vi "Generate Resampling Parameters.vi"(10 "X.ZOOM (Linear)":dbl, 11 "Stretch Array IN":dbl[](array[numeric])=[1.440619470870466, 1.4376467808189701, 1.4346907462529248, 1.431751260882534, 1.4288282193717416, 1.425921517328019, 1.4230310512922835, 1.4201567187289466, 1.4172984180160932, 1.4144560484357853, 1.4116295101644896, 1.4088187042636287, 1.4060235326702533, 1.4032438981878341, 1.4004797044771675, 1.397730856047402, 1.3949972582471741, 1.3922788172558593, 1.3895754400749307, 1.3868870345194306, 1.3842135092095456, 1.3815547735622893, 1.3789107377832892, 1.3762813128586768, 1.3736664105470766, 1.3710659433716992, 1.368479824612527, 1.3659079682986035, 1.3633502892004121, 1.3608067028223534, 1.3582771253953125, 1.3557614738693209, 1.3532596659063045, 1.3507716198729252, 1.348297254833506, 1.3458364905430458, 1.343389247440318, 1.3409554466410527, 1.3385350099312032, 1.3361278597602924, 1.3337339192348416, 1.3313531121118791, 1.328985362792523, 1.3266305963156464, 1.3242887383516175, 1.321959715196112, 1.3196434537640023, 1.3173398815833195, 1.3150489267892873, 1.3127705181184264, 1.3105045849027293, 1.308251057063904, 1.3060098651076884, 1.303780940118227, 1.301564213752519, 1.2993596182349283, 1.2971670863517617, 1.2949865514459058, 1.2928179474115327, 1.2906612086888616, 1.2885162702589879, 1.2863830676387666, 1.2842615368757604, 1.282151614543242, 1.2800532377352587, 1.2779663440617515, 1.2758908716437318, 1.2738267591085115, 1.2717739455849928, 1.2697323706990076, 1.2677019745687121, 1.2656826978000357, 1.2636744814821805, 1.261677267183171, 1.259690996945458, 1.25771561328157, 1.255751059169815, 1.2537972780500308, 1.251854213819384, 1.2499218108282157, 1.248000013875936, 1.2460887682069621, 1.2441880195067057, 1.2422977138976015, 1.2404177979351838, 1.2385482186042058, 1.236688923314801, 1.2348398598986912, 1.233000976605433, 1.2311722220987076, 1.2293535454526525, 1.2275448961482345, 1.2257462240696608, 1.2239574795008314, 1.2221786131218302, 1.2204095760054567, 1.2186503196137932, 1.2169007957948108, 1.2151609567790143, 1.2134307551761225, 1.2117101439717848, 1.2099990765243347, 1.2082975065615775, 1.2066053881776153, 1.204922675829705, 1.2032493243351499, 1.2015852888682272, 1.1999305249571475, 1.1982849884810485, 1.1966486356670185, 1.195021423087156, 1.1934033076556592, 1.1917942466259448, 1.1901941975878023, 1.188603118464577, 1.1870209675103802, 1.1854477033073352, 1.183883284762848, 1.18232767110691, 1.1807808218894282, 1.1792426969775847, 1.1777132565532245, 1.1761924611102694, 1.1746802714521631, 1.1731766486893391, 1.1716815542367196, 1.170194949811237, 1.1687167974293855, 1.1672470594047961, 1.1657856983458381, 1.1643326771532463, 1.1628879590177723, 1.1614515074178609, 1.1600232861173525, 1.1586032591632074, 1.1571913908832554, 1.155787645883968, 1.1543919890482561, 1.1530043855332879, 1.1516248007683323, 1.1502532004526227, 1.1488895505532448, 1.1475338173030458, 1.1461859671985648, 1.144845966997986, 1.1435137837191125, 1.1421893846373607, 1.1408727372837775, 1.1395638094430751, 1.138262569151689, 1.1369689846958546, 1.1356830246097043, 1.134404657673384, 1.1331338529111887, 1.131870579589719, 1.1306148072160556, 1.1293665055359505, 1.1281256445320416, 1.1268921944220818, 1.1256661256571876, 1.124447408920106, 1.1232360151234988, 1.1220319154082454, 1.1208350811417611, 1.1196454839163357, 1.1184630955474852, 1.1172878880723252, 1.1161198337479559, 1.1149589050498683, 1.1138050746703627, 1.1126583155169876, 1.1115186007109896, 1.1103859035857837, 1.1092601976854366, 1.108141456763167, 1.1070296547798593, 1.105924765902595, 1.104826764503197, 1.1037356251567896, 1.1026513226403736, 1.101573831931415, 1.100503128206449, 1.0994391868396975, 1.0983819834017015, 1.097331493657966, 1.0962876935676213, 1.0952505592820947, 1.0942200671437987, 1.0931961936848302, 1.0921789156256847, 1.091168209873983, 1.09016405352321, 1.0891664238514684, 1.0881752983202426, 1.0871906545731778, 1.0862124704348681, 1.0852407239096624, 1.0842753931804756, 1.083316456607618, 1.0823638927276333, 1.0814176802521487, 1.0804777980667386, 1.0795442252297975, 1.0786169409714261, 1.077695924692329, 1.0767811559627212, 1.075872614521249, 1.0749702802739198, 1.0740741332930437, 1.0731841538161861, 1.0723003222451302, 1.0714226191448506, 1.0705510252424983, 1.0696855214263945, 1.068826088745036, 1.067972708406111, 1.0671253617755228, 1.066284030376427, 1.0654486958882756, 1.0646193401458734, 1.0637959451384424, 1.0629784930086954, 1.0621669660519228, 1.0613613467150842, 1.060561617595912, 1.059767761442025, 1.0589797611500482, 1.0581975997647464, 1.0574212604781612, 1.0566507266287621, 1.0558859817006039, 1.0551270093224923, 1.0543737932671609, 1.0536263174504543, 1.052884565930521, 1.0521485229070153, 1.0514181727203058, 1.0506934998506943, 1.0499744889176423, 1.0492611246790045, 1.0485533920302719, 1.047851276003824, 1.0471547617681856, 1.0464638346272943, 1.0457784800197756, 1.0450986835182245, 1.0444244308284962, 1.0437557077890038, 1.0430925003700235, 1.0424347946730084, 1.0417825769299076, 1.0411358335024952, 1.0404945508817052, 1.039858715686974, 1.0392283146655907, 1.0386033346920531, 1.0379837627674322, 1.037369586018744, 1.036760791698327, 1.0361573671832274, 1.035559299974591, 1.0349665776970631, 1.034379188098192, 1.0337971190478439, 1.03322035853762, 1.0326488946802839, 1.0320827157091916, 1.0315218099777332, 1.0309661659587757, 1.0304157722441156, 1.029870617543938, 1.0293306906862798, 1.0287959806165006, 1.0282664763967595, 1.0277421672054998, 1.0272230423369366, 1.0267090912005525, 1.0262003033206, 1.025696668335608, 1.0251981759978956, 1.0247048161730927, 1.024216578839663, 1.0237334540884373, 1.023255432122149, 1.0227825032549778, 1.0223146579120976, 1.0218518866292314, 1.0213941800522104, 1.0209415289365391, 1.0204939241469677, 1.0200513566570675, 1.0196138175488132, 1.0191812980121713, 1.0187537893446912, 1.0183312829511053, 1.0179137703429328, 1.017501243138087, 1.0170936930604915, 1.016691111939699, 1.0162934917105162, 1.0159008244126346, 1.0155131021902641, 1.0151303172917756, 1.0147524620693449, 1.0143795289786035, 1.0140115105782945, 1.0136483995299344, 1.013290188597476, 1.012936870646982, 1.0125884386462984, 1.0122448856647361, 1.011906204872756, 1.0115723895416593, 1.0112434330432825, 1.0109193288496965, 1.0106000705329132, 1.0102856517645928, 1.0099760663157593, 1.0096713080565187, 1.009371370955783, 1.0090762490809977, 1.0087859365978757, 1.0085004277701342, 1.0082197169592362, 1.0079437986241382, 1.0076726673210412, 1.0074063177031463, 1.0071447445204138, 1.0068879426193307, 1.0066359069426771, 1.0063886325293019, 1.0061461145138997, 1.005908348126794, 1.005675328693725, 1.0054470516356384, 1.0052235124684836, 1.0050047068030135, 1.0047906303445873, 1.0045812788929813, 1.0043766483422008, 1.0041767346802974, 1.003981533989191, 1.0037910424444962, 1.003605256315351, 1.0034241719642527, 1.0032477858468958, 1.003076094512014, 1.0029090946012298, 1.0027467828489023, 1.0025891560819855, 1.0024362112198855, 1.0022879452743259, 1.0021443553492149, 1.0020054386405173, 1.00187119243613, 1.0017416141157636, 1.0016167011508252, 1.0014964511043074, 1.0013808616306805, 1.0012699304757895, 1.0011636554767542, 1.0010620345618735, 1.0009650657505351, 1.0008727471531271, 1.0007850769709556, 1.0007020534961644, 1.0006236751116613, 1.0005499402910454, 1.0004808475985407, 1.000416395688933, 1.0003565833075099, 1.0003014092900064, 1.0002508725625538, 1.000204972141631, 1.0001637071340235, 1.000127076736782, 1.0000950802371884, 1.000067717012724, 1.0000449865310421, 1.0000268883499448, 1.0000134221173627, 1.0000045875713393, 1.000000384540001, 1.0000008129417106, 1.0000058727846188, 1.00001556416725, 1.0000298872781128, 1.000048842395831, 1.0000724298891448, 1.000100650216928, 1.0001335039282069, 1.0001709916621842, 1.0002131141482686, 1.000259872206105, 1.0003112667456115, 1.00036729876702, 1.0004279693609184, 1.0004932797083008, 1.0005632310806174, 1.0006378248398318, 1.0007170624384805, 1.0008009454197369, 1.0008894754174789, 1.0009826541563618, 1.0010804834518927, 1.0011829652105122, 1.0012901014296773, 1.0014018941979497, 1.0015183456950882, 1.0016394581921442, 1.0017652340515628, 1.0018956757272859, 1.0020307857648618, 1.0021705668015566, 1.0023150215664711, 1.0024641528806615, 1.0026179636572636, 1.0027764569016226, 1.002939635711425, 1.0031075032768366, 1.0032800628806426, 1.003457317898394, 1.0036392717985572, 1.0038259281426667, 1.004017290585485, 1.0042133628751624, 1.0044141488534049, 1.0046196524556448, 1.0048298777112152, 1.0050448287435292, 1.0052645097702635, 1.005488925103546, 1.0057180791501472, 1.0059519764116787, 1.0061906214847909, 1.0064340190613805, 1.006682173928799, 1.0069350909700665, 1.0071927751640892, 1.0074552315858845, 1.0077224654068047, 1.007994481894772, 1.0082712864145116, 1.0085528844277947, 1.0088392814936815, 1.0091304832687726, 1.0094264955074617, 1.0097273240621956, 1.0100329748837367, 1.010343454021431, 1.0106587676234822, 1.0109789219372267, 1.0113039233094172, 1.011633778186509, 1.0119684931149513, 1.0123080747414843, 1.0126525298134386, 1.0130018651790424, 1.0133560877877317, 1.013715204690466, 1.0140792230400482, 1.0144481500914506, 1.014821993202145, 1.0152007598324373, 1.0155844575458093, 1.0159730940092622, 1.016366676993668, 1.016765214374125, 1.0171687141303176, 1.0175771843468828, 1.017990633213781, 1.0184090690266712, 1.0188325001872929, 1.0192609352038535, 1.019694382691419, 1.020132851372312, 1.0205763500765135, 1.0210248877420718, 1.021478473415516, 1.0219371162522737, 1.022400825517097, 1.022869610584492, 1.0233434809391537, 1.0238224461764078, 1.0243065160026579, 1.0247957002358377, 1.025290008805869, 1.0257894517551263, 1.0262940392389066, 1.026803781525905, 1.0273186889986967, 1.0278387721542241, 1.0283640416042907, 1.0288945080760612, 1.029430182412566, 1.029971075573214, 1.0305171986343111, 1.031068562789582, 1.0316251793507032, 1.0321870597478386, 1.0327542155301825, 1.0333266583665095, 1.0339044000457294, 1.0344874524774512, 1.0350758276925507, 1.0356695378437466, 1.036268595206182, 1.0368730121780148, 1.0374828012810111, 1.0380979751611497, 1.03871854658923, 1.039344528461488]) -> (2 "Modified Midpoint pixel (After stretch)":i32, 3 "Window size and Resampling OUT":T1(array[cluster]))   [LabVIEW 2012]
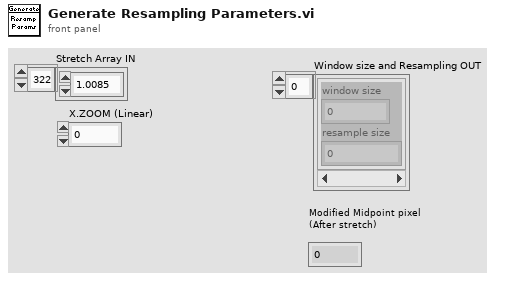
[diagram p1: front panel]
types:
  T1 = cluster{"window size":i32, "resample size":i32}[]
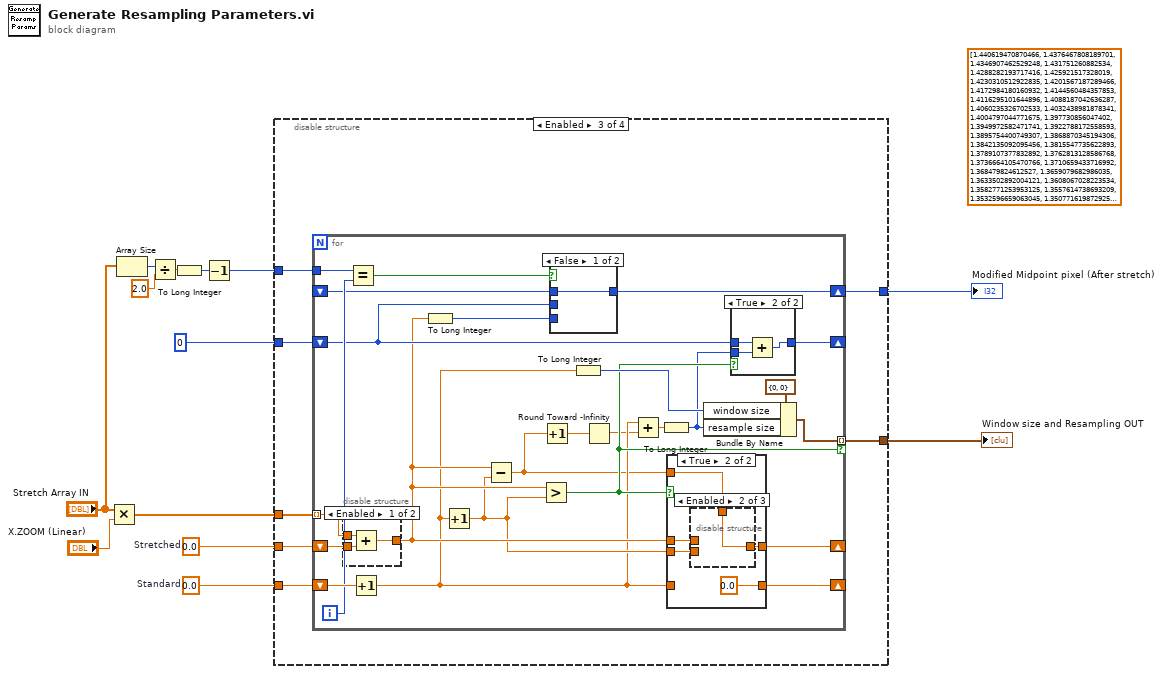
[diagram p0: block diagram]
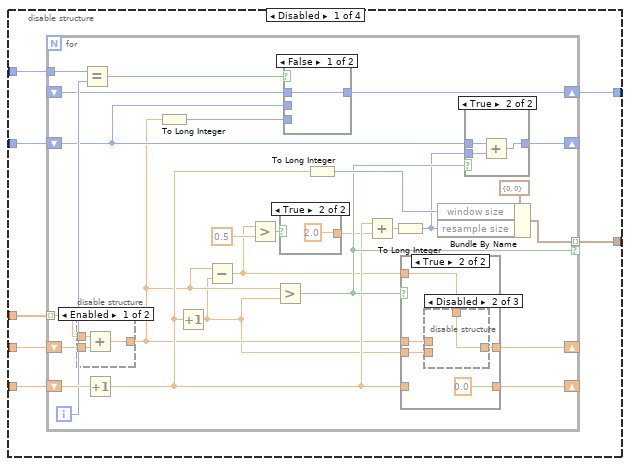
[diagram p2: hidden frame]
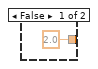
[diagram p3: hidden frame]
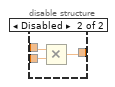
[diagram p4: hidden frame]
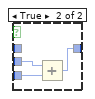
[diagram p5: hidden frame]
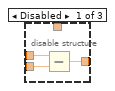
[diagram p8: hidden frame]
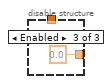
[diagram p9: hidden frame]
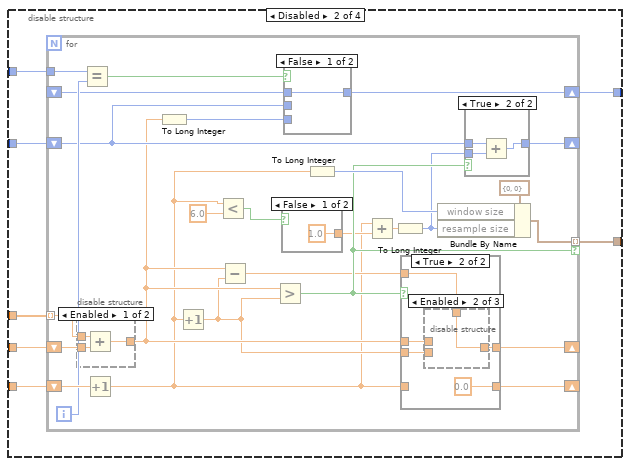
[diagram p10: hidden frame]
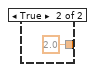
[diagram p11: hidden frame]
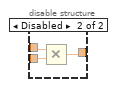
[diagram p12: hidden frame]
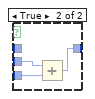
[diagram p13: hidden frame]
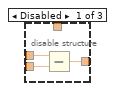
[diagram p16: hidden frame]
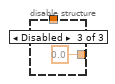
[diagram p17: hidden frame]
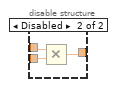
[diagram p18: hidden frame]
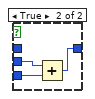
[diagram p19: hidden frame]
diagram:
  w12 = 0.0  # Stretched
  w13 = 0.0  # Standard
  (unwired) dbl[] [1.440619470870466, 1.4376467808189701, 1.4346907462529248, 1.431751260882534, 1.4288282193717416, 1.425921517328019, 1.4230310512922835, 1.4201567187289466, 1.4172984180160932, 1.4144560484357853, 1.4116295101644896, 1.4088187042636287, 1.4060235326702533, 1.4032438981878341, 1.4004797044771675, 1.397730856047402, 1.3949972582471741, 1.3922788172558593, 1.3895754400749307, 1.3868870345194306, 1.3842135092095456, 1.3815547735622893, 1.3789107377832892, 1.3762813128586768, 1.3736664105470766, 1.3710659433716992, 1.368479824612527, 1.3659079682986035, 1.3633502892004121, 1.3608067028223534, 1.3582771253953125, 1.3557614738693209, 1.3532596659063045, 1.3507716198729252, 1.348297254833506, 1.3458364905430458, 1.343389247440318, 1.3409554466410527, 1.3385350099312032, 1.3361278597602924, 1.3337339192348416, 1.3313531121118791, 1.328985362792523, 1.3266305963156464, 1.3242887383516175, 1.321959715196112, 1.3196434537640023, 1.3173398815833195, 1.3150489267892873, 1.3127705181184264, 1.3105045849027293, 1.308251057063904, 1.3060098651076884, 1.303780940118227, 1.301564213752519, 1.2993596182349283, 1.2971670863517617, 1.2949865514459058, 1.2928179474115327, 1.2906612086888616, 1.2885162702589879, 1.2863830676387666, 1.2842615368757604, 1.282151614543242, 1.2800532377352587, 1.2779663440617515, 1.2758908716437318, 1.2738267591085115, 1.2717739455849928, 1.2697323706990076, 1.2677019745687121, 1.2656826978000357, 1.2636744814821805, 1.261677267183171, 1.259690996945458, 1.25771561328157, 1.255751059169815, 1.2537972780500308, 1.251854213819384, 1.2499218108282157, 1.248000013875936, 1.2460887682069621, 1.2441880195067057, 1.2422977138976015, 1.2404177979351838, 1.2385482186042058, 1.236688923314801, 1.2348398598986912, 1.233000976605433, 1.2311722220987076, 1.2293535454526525, 1.2275448961482345, 1.2257462240696608, 1.2239574795008314, 1.2221786131218302, 1.2204095760054567, 1.2186503196137932, 1.2169007957948108, 1.2151609567790143, 1.2134307551761225, 1.2117101439717848, 1.2099990765243347, 1.2082975065615775, 1.2066053881776153, 1.204922675829705, 1.2032493243351499, 1.2015852888682272, 1.1999305249571475, 1.1982849884810485, 1.1966486356670185, 1.195021423087156, 1.1934033076556592, 1.1917942466259448, 1.1901941975878023, 1.188603118464577, 1.1870209675103802, 1.1854477033073352, 1.183883284762848, 1.18232767110691, 1.1807808218894282, 1.1792426969775847, 1.1777132565532245, 1.1761924611102694, 1.1746802714521631, 1.1731766486893391, 1.1716815542367196, 1.170194949811237, 1.1687167974293855, 1.1672470594047961, 1.1657856983458381, 1.1643326771532463, 1.1628879590177723, 1.1614515074178609, 1.1600232861173525, 1.1586032591632074, 1.1571913908832554, 1.155787645883968, 1.1543919890482561, 1.1530043855332879, 1.1516248007683323, 1.1502532004526227, 1.1488895505532448, 1.1475338173030458, 1.1461859671985648, 1.144845966997986, 1.1435137837191125, 1.1421893846373607, 1.1408727372837775, 1.1395638094430751, 1.138262569151689, 1.1369689846958546, 1.1356830246097043, 1.134404657673384, 1.1331338529111887, 1.131870579589719, 1.1306148072160556, 1.1293665055359505, 1.1281256445320416, 1.1268921944220818, 1.1256661256571876, 1.124447408920106, 1.1232360151234988, 1.1220319154082454, 1.1208350811417611, 1.1196454839163357, 1.1184630955474852, 1.1172878880723252, 1.1161198337479559, 1.1149589050498683, 1.1138050746703627, 1.1126583155169876, 1.1115186007109896, 1.1103859035857837, 1.1092601976854366, 1.108141456763167, 1.1070296547798593, 1.105924765902595, 1.104826764503197, 1.1037356251567896, 1.1026513226403736, 1.101573831931415, 1.100503128206449, 1.0994391868396975, 1.0983819834017015, 1.097331493657966, 1.0962876935676213, 1.0952505592820947, 1.0942200671437987, 1.0931961936848302, 1.0921789156256847, 1.091168209873983, 1.09016405352321, 1.0891664238514684, 1.0881752983202426, 1.0871906545731778, 1.0862124704348681, 1.0852407239096624, 1.0842753931804756, 1.083316456607618, 1.0823638927276333, 1.0814176802521487, 1.0804777980667386, 1.0795442252297975, 1.0786169409714261, 1.077695924692329, 1.0767811559627212, 1.075872614521249, 1.0749702802739198, 1.0740741332930437, 1.0731841538161861, 1.0723003222451302, 1.0714226191448506, 1.0705510252424983, 1.0696855214263945, 1.068826088745036, 1.067972708406111, 1.0671253617755228, 1.066284030376427, 1.0654486958882756, 1.0646193401458734, 1.0637959451384424, 1.0629784930086954, 1.0621669660519228, 1.0613613467150842, 1.060561617595912, 1.059767761442025, 1.0589797611500482, 1.0581975997647464, 1.0574212604781612, 1.0566507266287621, 1.0558859817006039, 1.0551270093224923, 1.0543737932671609, 1.0536263174504543, 1.052884565930521, 1.0521485229070153, 1.0514181727203058, 1.0506934998506943, 1.0499744889176423, 1.0492611246790045, 1.0485533920302719, 1.047851276003824, 1.0471547617681856, 1.0464638346272943, 1.0457784800197756, 1.0450986835182245, 1.0444244308284962, 1.0437557077890038, 1.0430925003700235, 1.0424347946730084, 1.0417825769299076, 1.0411358335024952, 1.0404945508817052, 1.039858715686974, 1.0392283146655907, 1.0386033346920531, 1.0379837627674322, 1.037369586018744, 1.036760791698327, 1.0361573671832274, 1.035559299974591, 1.0349665776970631, 1.034379188098192, 1.0337971190478439, 1.03322035853762, 1.0326488946802839, 1.0320827157091916, 1.0315218099777332, 1.0309661659587757, 1.0304157722441156, 1.029870617543938, 1.0293306906862798, 1.0287959806165006, 1.0282664763967595, 1.0277421672054998, 1.0272230423369366, 1.0267090912005525, 1.0262003033206, 1.025696668335608, 1.0251981759978956, 1.0247048161730927, 1.024216578839663, 1.0237334540884373, 1.023255432122149, 1.0227825032549778, 1.0223146579120976, 1.0218518866292314, 1.0213941800522104, 1.0209415289365391, 1.0204939241469677, 1.0200513566570675, 1.0196138175488132, 1.0191812980121713, 1.0187537893446912, 1.0183312829511053, 1.0179137703429328, 1.017501243138087, 1.0170936930604915, 1.016691111939699, 1.0162934917105162, 1.0159008244126346, 1.0155131021902641, 1.0151303172917756, 1.0147524620693449, 1.0143795289786035, 1.0140115105782945, 1.0136483995299344, 1.013290188597476, 1.012936870646982, 1.0125884386462984, 1.0122448856647361, 1.011906204872756, 1.0115723895416593, 1.0112434330432825, 1.0109193288496965, 1.0106000705329132, 1.0102856517645928, 1.0099760663157593, 1.0096713080565187, 1.009371370955783, 1.0090762490809977, 1.0087859365978757, 1.0085004277701342, 1.0082197169592362, 1.0079437986241382, 1.0076726673210412, 1.0074063177031463, 1.0071447445204138, 1.0068879426193307, 1.0066359069426771, 1.0063886325293019, 1.0061461145138997, 1.005908348126794, 1.005675328693725, 1.0054470516356384, 1.0052235124684836, 1.0050047068030135, 1.0047906303445873, 1.0045812788929813, 1.0043766483422008, 1.0041767346802974, 1.003981533989191, 1.0037910424444962, 1.003605256315351, 1.0034241719642527, 1.0032477858468958, 1.003076094512014, 1.0029090946012298, 1.0027467828489023, 1.0025891560819855, 1.0024362112198855, 1.0022879452743259, 1.0021443553492149, 1.0020054386405173, 1.00187119243613, 1.0017416141157636, 1.0016167011508252, 1.0014964511043074, 1.0013808616306805, 1.0012699304757895, 1.0011636554767542, 1.0010620345618735, 1.0009650657505351, 1.0008727471531271, 1.0007850769709556, 1.0007020534961644, 1.0006236751116613, 1.0005499402910454, 1.0004808475985407, 1.000416395688933, 1.0003565833075099, 1.0003014092900064, 1.0002508725625538, 1.000204972141631, 1.0001637071340235, 1.000127076736782, 1.0000950802371884, 1.000067717012724, 1.0000449865310421, 1.0000268883499448, 1.0000134221173627, 1.0000045875713393, 1.000000384540001, 1.0000008129417106, 1.0000058727846188, 1.00001556416725, 1.0000298872781128, 1.000048842395831, 1.0000724298891448, 1.000100650216928, 1.0001335039282069, 1.0001709916621842, 1.0002131141482686, 1.000259872206105, 1.0003112667456115, 1.00036729876702, 1.0004279693609184, 1.0004932797083008, 1.0005632310806174, 1.0006378248398318, 1.0007170624384805, 1.0008009454197369, 1.0008894754174789, 1.0009826541563618, 1.0010804834518927, 1.0011829652105122, 1.0012901014296773, 1.0014018941979497, 1.0015183456950882, 1.0016394581921442, 1.0017652340515628, 1.0018956757272859, 1.0020307857648618, 1.0021705668015566, 1.0023150215664711, 1.0024641528806615, 1.0026179636572636, 1.0027764569016226, 1.002939635711425, 1.0031075032768366, 1.0032800628806426, 1.003457317898394, 1.0036392717985572, 1.0038259281426667, 1.004017290585485, 1.0042133628751624, 1.0044141488534049, 1.0046196524556448, 1.0048298777112152, 1.0050448287435292, 1.0052645097702635, 1.005488925103546, 1.0057180791501472, 1.0059519764116787, 1.0061906214847909, 1.0064340190613805, 1.006682173928799, 1.0069350909700665, 1.0071927751640892, 1.0074552315858845, 1.0077224654068047, 1.007994481894772, 1.0082712864145116, 1.0085528844277947, 1.0088392814936815, 1.0091304832687726, 1.0094264955074617, 1.0097273240621956, 1.0100329748837367, 1.010343454021431, 1.0106587676234822, 1.0109789219372267, 1.0113039233094172, 1.011633778186509, 1.0119684931149513, 1.0123080747414843, 1.0126525298134386, 1.0130018651790424, 1.0133560877877317, 1.013715204690466, 1.0140792230400482, 1.0144481500914506, 1.014821993202145, 1.0152007598324373, 1.0155844575458093, 1.0159730940092622, 1.016366676993668, 1.016765214374125, 1.0171687141303176, 1.0175771843468828, 1.017990633213781, 1.0184090690266712, 1.0188325001872929, 1.0192609352038535, 1.019694382691419, 1.020132851372312, 1.0205763500765135, 1.0210248877420718, 1.021478473415516, 1.0219371162522737, 1.022400825517097, 1.022869610584492, 1.0233434809391537, 1.0238224461764078, 1.0243065160026579, 1.0247957002358377, 1.025290008805869, 1.0257894517551263, 1.0262940392389066, 1.026803781525905, 1.0273186889986967, 1.0278387721542241, 1.0283640416042907, 1.0288945080760612, 1.029430182412566, 1.029971075573214, 1.0305171986343111, 1.031068562789582, 1.0316251793507032, 1.0321870597478386, 1.0327542155301825, 1.0333266583665095, 1.0339044000457294, 1.0344874524774512, 1.0350758276925507, 1.0356695378437466, 1.036268595206182, 1.0368730121780148, 1.0374828012810111, 1.0380979751611497, 1.03871854658923, 1.039344528461488]
  n1 = Multiply(x="Stretch Array IN", y="X.ZOOM (Linear)") -> (x*y=w9:dbl[])
  n2 = Array Size(array="Stretch Array IN") -> (size(s)=w7:i32)
  n3 = Divide(x=w7, y=2.0) -> (x/y=w5:dbl)
  n4 = To Long Integer(number=w5) -> (32bit integer=w4:i32)
  n5 = Decrement(x=w4) -> (x-1=w3:i32)
  n6 = disable-structure shown="Enabled" {
    disable-tunnel: w13 -> [w20 w81 w142 _]
    disable-tunnel: w12 -> [w19 w80 w141 _]
    disable-tunnel: [w18 w79 w140 _] -> w11
    disable-tunnel: w9 -> [w17 w78 w139 _]
    disable-tunnel: w3 -> [w16 w77 w138 _]
    disable-tunnel: 0 -> [w15 w76 w137 _]
    disable-tunnel: [w14 w75 w136 _] -> w1
    frame Disabled {
      n7 = for {
        tunnel: w17 -> [w46] mode=indexing
        shift-right: [w42] -> _
        shift-left: w20 -> [w44]
        shift-right: [w43] -> _
        shift-left: w19 -> [w45]
        tunnel: [w40] -> w18 mode=indexing if=w36
        tunnel: w16 -> [w38]
        shift-right: [w34] -> _
        shift-left: w15 -> [w32]
        shift-right: [w30] -> w14
        shift-left: _ -> [w29]
        i -> [w37]
        n8 = disable-structure shown="Enabled" {
          disable-tunnel: w46 -> [w51 w54]
          disable-tunnel: w45 -> [w50 w53]
          disable-tunnel: [w49 w52] -> w25
          frame Enabled {
            n9 = Add(x=w51, y=w50) -> (x+y=w49:dbl)
          }
          frame Disabled {
            n10 = Multiply(x=w54, y=w53) -> (x*y=w52:dbl)
          }
        }
        n11 = Equal?(x=w38, y=w37) -> (x = y?=w33:bool)
        n12 = Increment(x=w44) -> (x+1=w28:dbl)
        n13 = To Long Integer(number=w25) -> (32bit integer=w31:i32)
        n14 = Increment(x=w28) -> (x+1=w24:dbl)
        n15 = Subtract(x=w25, y=w24) -> (x-y=w21:dbl)
        n16 = Greater?(x=w21, y=0.5) -> (0:w22:bool)
        n17 = Greater?(x=w25, y=w24) -> (0:w36:bool)
        n18 = case shown="True" w22 {
          tunnel: [2.0 ("y") 2.0 ("y")] -> w27
          frame False {
          }
          frame True {
          }
        }
        n19 = case shown="False" w33 {
          tunnel: w32 -> [_ w58]
          tunnel: w31 -> [_ w57]
          tunnel: [w55 w56] -> w30
          tunnel: w29 -> [w55 _]
          frame False {
          }
          frame True {
            n20 = Add(x=w58, y=w57) -> (x+y=w56:i32)
          }
        }
        n21 = To Long Integer(number=w28) -> (32bit integer=w39:i32)
        n22 = Add(x=w28, y=w27) -> (x+y=w26:dbl)
        n23 = To Long Integer(number=w26) -> (32bit integer=w35:i32)
        n24 = case shown="True" w36 {
          tunnel: w28 -> [w63 _]
          tunnel: w25 -> [w64 w68]
          tunnel: [w64 w66] -> w43
          tunnel: [w63 0.0] -> w42
          tunnel: w24 -> [_ w67]
          tunnel: w21 -> [_ w65]
          frame False {
          }
          frame True {
            n25 = disable-structure shown="Disabled" {
              disable-tunnel: w68 -> [w72 _ _]
              disable-tunnel: w67 -> [w71 _ _]
              disable-tunnel: [w70 w73 0.0] -> w66
              disable-tunnel: w65 -> [_ w73 _]
              frame Disabled {
                n26 = Subtract(x=w72, y=w71) -> (x-y=w70:dbl)
              }
              frame Disabled {
              }
              frame Enabled {
              }
            }
          }
        }
        n27 = Bundle By Name(cluster=cluster{"window size":i32, "resample size":i32} {"window size"=0, "resample size"=0}, "window size"=w39, "resample size"=w35) -> (w40:cluster{"window size":i32, "resample size":i32})
        n28 = case shown="True" w36 {
          tunnel: w32 -> [w59 w62]
          tunnel: w35 -> [_ w61]
          tunnel: [w59 w60] -> w34
          frame False {
          }
          frame True {
            n29 = Add(x=w62, y=w61) -> (x+y=w60:i32)
          }
        }
      }
    }
    frame Disabled {
      n30 = for {
        tunnel: w78 -> [w107] mode=indexing
        shift-right: [w103] -> _
        shift-left: w81 -> [w105]
        shift-right: [w104] -> _
        shift-left: w80 -> [w106]
        tunnel: [w101] -> w79 mode=indexing if=w97
        tunnel: w77 -> [w99]
        shift-right: [w95] -> _
        shift-left: w76 -> [w93]
        shift-right: [w91] -> w75
        shift-left: _ -> [w90]
        i -> [w98]
        n31 = disable-structure shown="Enabled" {
          disable-tunnel: w107 -> [w112 w115]
          disable-tunnel: w106 -> [w111 w114]
          disable-tunnel: [w110 w113] -> w87
          frame Enabled {
            n32 = Add(x=w112, y=w111) -> (x+y=w110:dbl)
          }
          frame Disabled {
            n33 = Multiply(x=w115, y=w114) -> (x*y=w113:dbl)
          }
        }
        n34 = Equal?(x=w99, y=w98) -> (x = y?=w94:bool)
        n35 = Increment(x=w105) -> (x+1=w84:dbl)
        n36 = To Long Integer(number=w87) -> (32bit integer=w92:i32)
        n37 = Increment(x=w84) -> (x+1=w85:dbl)
        n38 = Less?(x=w84, y=6.0) -> (x < y?=w82:bool)
        n39 = Subtract(x=w87, y=w85) -> (x-y=w86:dbl)
        n40 = Greater?(x=w87, y=w85) -> (0:w97:bool)
        n41 = case shown="False" w82 {
          tunnel: [1.0 ("y") 2.0 ("y")] -> w89
          frame False {
          }
          frame True {
          }
        }
        n42 = case shown="False" w94 {
          tunnel: w93 -> [_ w119]
          tunnel: w92 -> [_ w118]
          tunnel: [w116 w117] -> w91
          tunnel: w90 -> [w116 _]
          frame False {
          }
          frame True {
            n43 = Add(x=w119, y=w118) -> (x+y=w117:i32)
          }
        }
        n44 = To Long Integer(number=w84) -> (32bit integer=w100:i32)
        n45 = Add(x=w84, y=w89) -> (x+y=w88:dbl)
        n46 = To Long Integer(number=w88) -> (32bit integer=w96:i32)
        n47 = case shown="True" w97 {
          tunnel: w84 -> [w124 _]
          tunnel: w87 -> [w125 w129]
          tunnel: [w125 w127] -> w104
          tunnel: [w124 0.0] -> w103
          tunnel: w85 -> [_ w128]
          tunnel: w86 -> [_ w126]
          frame False {
          }
          frame True {
            n48 = disable-structure shown="Enabled" {
              disable-tunnel: w129 -> [w133 _ _]
              disable-tunnel: w128 -> [w132 _ _]
              disable-tunnel: [w131 w134 0.0] -> w127
              disable-tunnel: w126 -> [_ w134 _]
              frame Disabled {
                n49 = Subtract(x=w133, y=w132) -> (x-y=w131:dbl)
              }
              frame Enabled {
              }
              frame Disabled {
              }
            }
          }
        }
        n50 = Bundle By Name(cluster=cluster{"window size":i32, "resample size":i32} {"window size"=0, "resample size"=0}, "window size"=w100, "resample size"=w96) -> (w101:cluster{"window size":i32, "resample size":i32})
        n51 = case shown="True" w97 {
          tunnel: w93 -> [w120 w123]
          tunnel: w96 -> [_ w122]
          tunnel: [w120 w121] -> w95
          frame False {
          }
          frame True {
            n52 = Add(x=w123, y=w122) -> (x+y=w121:i32)
          }
        }
      }
    }
    frame Enabled {
      n53 = for {
        tunnel: w139 -> [w167] mode=indexing
        shift-right: [w163] -> _
        shift-left: w142 -> [w165]
        shift-right: [w164] -> _
        shift-left: w141 -> [w166]
        tunnel: [w161] -> w140 mode=indexing if=w157
        tunnel: w138 -> [w159]
        shift-right: [w155] -> _
        shift-left: w137 -> [w153]
        shift-right: [w151] -> w136
        shift-left: _ -> [w150]
        i -> [w158]
        n54 = disable-structure shown="Enabled" {
          disable-tunnel: w167 -> [w170 w173]
          disable-tunnel: w166 -> [w169 w172]
          disable-tunnel: [w168 w171] -> w148
          frame Enabled {
            n55 = Add(x=w170, y=w169) -> (x+y=w168:dbl)
          }
          frame Disabled {
            n56 = Multiply(x=w173, y=w172) -> (x*y=w171:dbl)
          }
        }
        n57 = Equal?(x=w159, y=w158) -> (x = y?=w154:bool)
        n58 = Increment(x=w165) -> (x+1=w146:dbl)
        n59 = To Long Integer(number=w148) -> (32bit integer=w152:i32)
        n60 = Increment(x=w146) -> (x+1=w147:dbl)
        n61 = Subtract(x=w148, y=w147) -> (x-y=w145:dbl)
        n62 = Greater?(x=w148, y=w147) -> (0:w157:bool)
        n63 = Increment(x=w145) -> (x+1=w144:dbl)
        n64 = case shown="False" w154 {
          tunnel: w153 -> [_ w177]
          tunnel: w152 -> [_ w176]
          tunnel: [w174 w175] -> w151
          tunnel: w150 -> [w174 _]
          frame False {
          }
          frame True {
            n65 = Add(x=w177, y=w176) -> (x+y=w175:i32)
          }
        }
        n66 = To Long Integer(number=w146) -> (32bit integer=w160:i32)
        n67 = Round Toward -Infinity(1:w144) -> (0:w143:dbl)
        n68 = Add(x=w146, y=w143) -> (x+y=w149:dbl)
        n69 = To Long Integer(number=w149) -> (32bit integer=w156:i32)
        n70 = case shown="True" w157 {
          tunnel: w146 -> [w182 _]
          tunnel: w148 -> [w183 w187]
          tunnel: [w183 w185] -> w164
          tunnel: [w182 0.0] -> w163
          tunnel: w147 -> [_ w186]
          tunnel: w145 -> [_ w184]
          frame False {
          }
          frame True {
            n71 = disable-structure shown="Enabled" {
              disable-tunnel: w187 -> [w191 _ _]
              disable-tunnel: w186 -> [w190 _ _]
              disable-tunnel: [w189 w192 0.0] -> w185
              disable-tunnel: w184 -> [_ w192 _]
              frame Disabled {
                n72 = Subtract(x=w191, y=w190) -> (x-y=w189:dbl)
              }
              frame Enabled {
              }
              frame Disabled {
              }
            }
          }
        }
        n73 = Bundle By Name(cluster=cluster{"window size":i32, "resample size":i32} {"window size"=0, "resample size"=0}, "window size"=w160, "resample size"=w156) -> (w161:cluster{"window size":i32, "resample size":i32})
        n74 = case shown="True" w157 {
          tunnel: w153 -> [w178 w181]
          tunnel: w156 -> [_ w180]
          tunnel: [w178 w179] -> w155
          frame False {
          }
          frame True {
            n75 = Add(x=w181, y=w180) -> (x+y=w179:i32)
          }
        }
      }
    }
    frame Disabled {
    }
  }
  "Window size and Resampling OUT" <- w11
  "Modified Midpoint pixel (After stretch)" <- w1
